vi "Auth Async.vi"(4 "Failed Response":refnum<class "Response.lvclass">, 6 "Complete Response":refnum<class "Response.lvclass">, 7 "Refresh Only?":bool, 9 "Timeout S":dbl=60.0, 10 "Async Authorization":refnum<class "Async Authorization.lvclass">, 11 "OAuth2 in":refnum<class "OAuth2.lvclass">) -> ()   [LabVIEW 2020, in "OAuth2.lvlib" / "OAuth2.lvclass"]
uses:
  OAuth2.lvclass
  OAuth2.lvclass/OAuth2.ctl
  Async Auth State.ctl
  OAuth2.lvlib
  lv-http-util/HTTP Utils/Request/Request.lvclass
  Async Authorization/Async Authorization.lvclass
  Request/Request.lvclass
  <vilib>/httpClient/LabVIEWHTTPClient.lvlib
  <vilib>/httpClient/POSTBuffer.vi
  lv-http-util/HTTP Utils/Response/Response.lvclass
  <vilib>/Platform/browser.llb/Open URL in Default Browser (string).vi
panel:
  out "Request URL":string
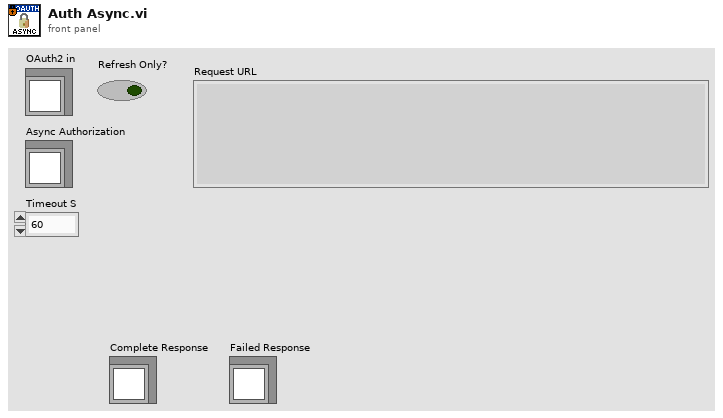
[diagram p1: front panel]
types:
  T1 = typedef "OAuth2.lvlib/Async Auth State.ctl" = enum16{"Initialize", "Request", "WaitAuth", "GetToken", "RefreshToken", "Complete", "Failed"}
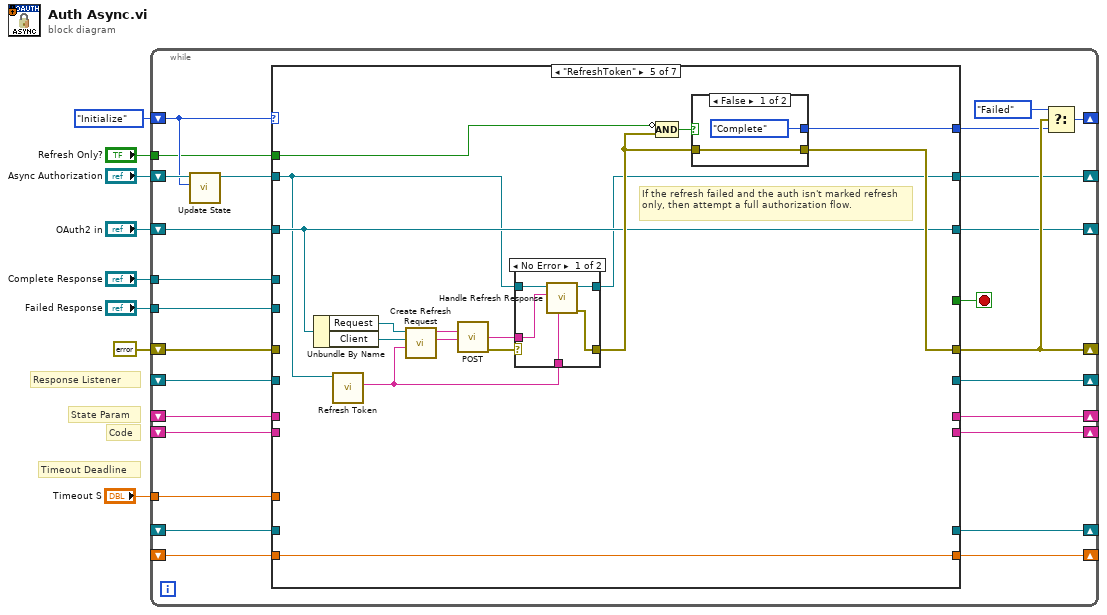
[diagram p0: block diagram]
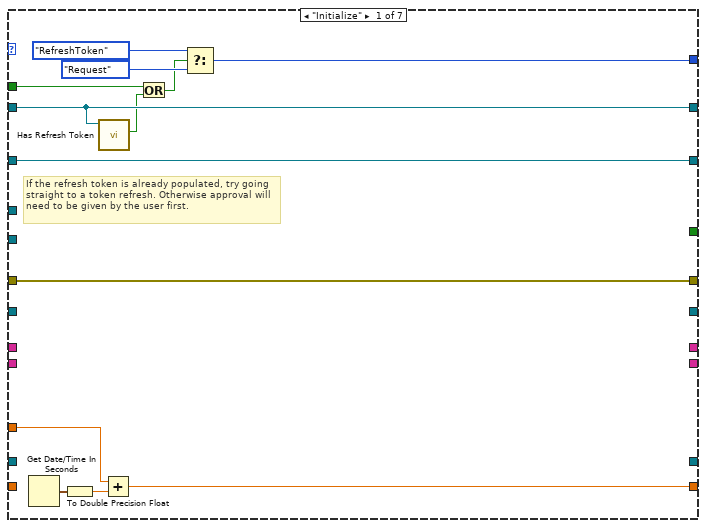
[diagram p2: hidden frame]
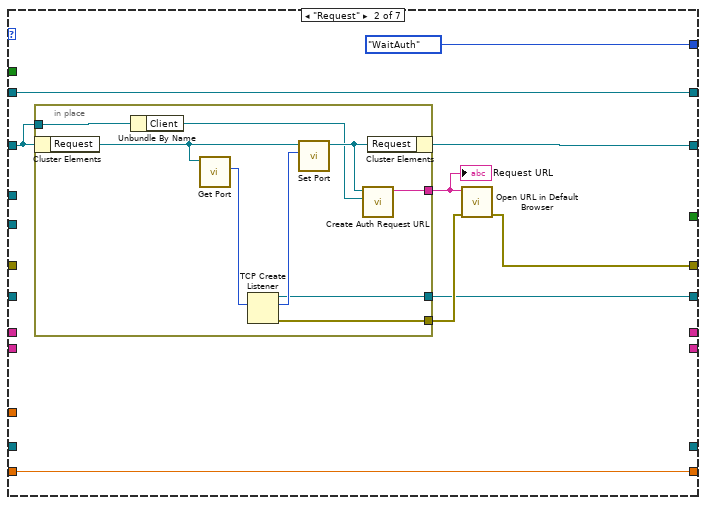
[diagram p3: hidden frame]
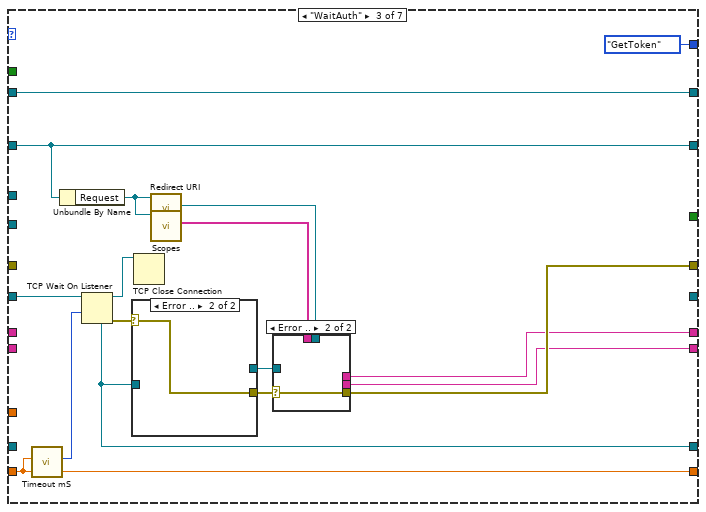
[diagram p4: hidden frame]
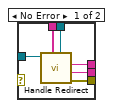
[diagram p5: hidden frame]
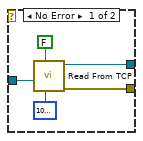
[diagram p6: hidden frame]
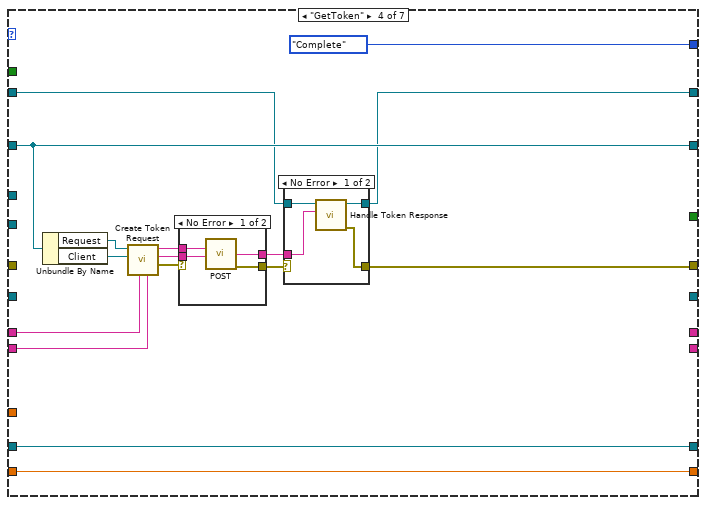
[diagram p7: hidden frame]
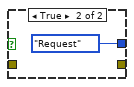
[diagram p10: hidden frame]
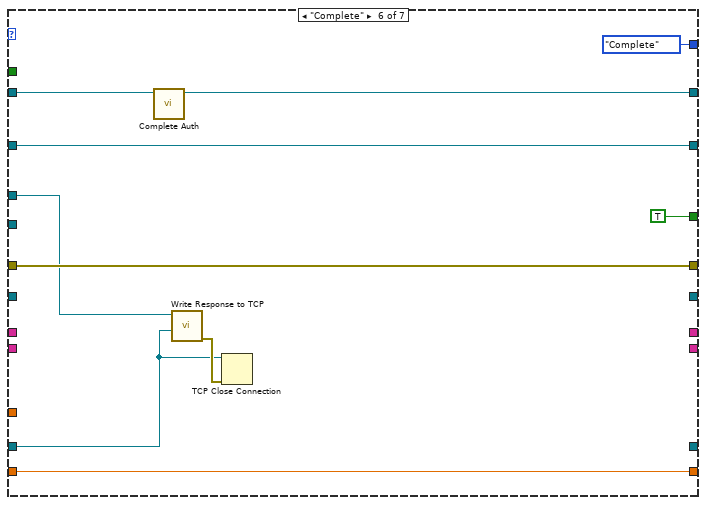
[diagram p12: hidden frame]
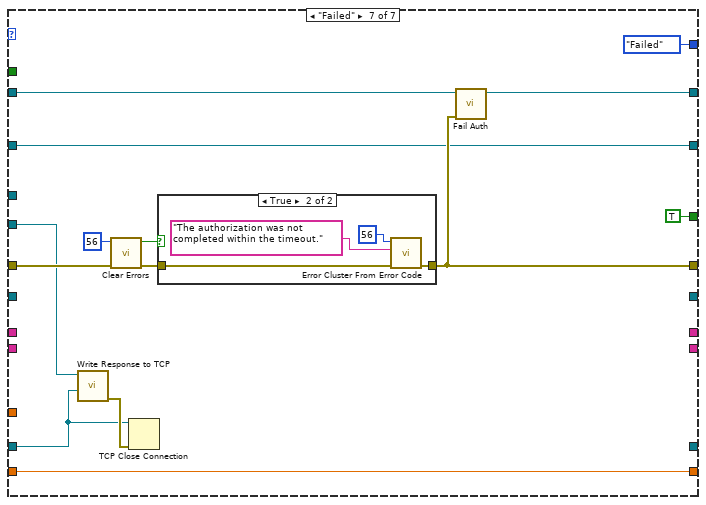
[diagram p13: hidden frame]
diagram:
  # "Timeout Deadline"
  # "Code"
  # "State Param"
  # "Response Listener"
  n1 = while {
    shift-right: [w18] -> _
    shift-left: Async_Auth_State."Initialize" ("State") -> [w28]
    shift-right: [w32] -> _
    shift-left: "OAuth2 in" -> [w33]
    shift-right: [w27] -> _
    shift-left: _ -> [w31]
    shift-right: [w26] -> _
    shift-left: _ -> [w24]
    shift-right: [w25] -> _
    shift-left: _ -> [w23]
    tunnel: "Timeout S" -> [w22]
    shift-right: [w21] -> _
    shift-left: _ -> [w20]
    shift-right: [w34] -> _
    shift-left: errorcluster {"status"=FALSE, "code"=0, "source"=""} ("error out") -> [w19]
    shift-right: [w15] -> _
    shift-left: "Async Authorization" -> [w30]
    tunnel: "Complete Response" -> [w13]
    tunnel: "Failed Response" -> [w12]
    shift-right: [w11] -> _
    shift-left: _ -> [w10]
    tunnel: "Refresh Only?" -> [w9]
    stop <- w14 stop-if-true
    n2 = call "Update State.vi"("Async Auth State"=w28, "Async Authorization in"=w30) -> ("Async Authorization out"=w29:refnum<class "Async Authorization.lvclass">)  [unwired: 9 in]
    n3 = case shown="\"RefreshToken\"" w28 {
      tunnel: w33 -> [w47 w54 w69 w111 w133 w152 w169]
      tunnel: [w47 w52 w69 w111 w133 w152 w169] -> w32
      tunnel: w31 -> [_ _ w81 _ _ _ _]
      tunnel: w29 -> [w39 w48 w76 w97 w127 w153 w167]
      tunnel: [_ w55 _ _ _ _ _] -> w27
      tunnel: [_ _ w71 _ _ _ _] -> w26
      tunnel: [_ _ w70 _ _ _ _] -> w25
      tunnel: w24 -> [_ _ _ w108 _ _ _]
      tunnel: w23 -> [_ _ _ w107 _ _ _]
      tunnel: w22 -> [w42 _ _ _ _ _ _]
      tunnel: [w41 w50 w80 w103 w136 w157 w168] -> w21
      tunnel: w20 -> [_ w50 w80 w103 w136 w157 w168]
      tunnel: [w38 w51 w72 w100 w138 w155 w171] -> w34
      tunnel: w19 -> [w38 _ _ _ _ w155 w172]
      tunnel: [w40 Async_Auth_State."WaitAuth" ("State") Async_Auth_State."GetToken" ("f") Async_Auth_State."Complete" ("f") w124 Async_Auth_State."Complete" ("f") Async_Auth_State."Failed" ("f")] -> w16
      tunnel: [w39 w48 w76 w98 w128 w151 w166] -> w15
      tunnel: [_ _ _ _ _ TRUE TRUE] -> w14
      tunnel: w13 -> [_ _ _ _ _ w149 _]
      tunnel: w12 -> [_ _ _ _ _ _ w163]
      tunnel: [_ _ w75 w96 _ _ _] -> w11
      tunnel: w10 -> [_ _ _ w96 _ w150 w162]
      tunnel: w9 -> [w37 _ _ _ w125 _ _]
      frame "Initialize" {
        # "If the refresh token is already populated, try going straight to a token refresh. Otherwise approval will need to be given by the user first."
        n4 = Get Date/Time In Seconds() -> (seconds since 1Jan1904=w44:timestamp)
        n5 = To Double Precision Float(number=w44) -> (double precision float=w43:dbl)
        n6 = call "Has Refresh Token.vi"("Async Authorization in"=w39) -> ("Has Refresh Token"=w36:bool)  [unwired: 10 in]
        n7 = Add(x=w42, y=w43) -> (x+y=w41:dbl)
        n8 = Or(x=w37, y=w36) -> (x .or. y?=w35:bool)
        n9 = Select(t=Async_Auth_State."RefreshToken" ("State"), s=w35, f=Async_Auth_State."Request") -> (s? t:f=w40:T1)
      }
      frame "Request" {
        n10 = in-place {
          in-place-border: [w63] -> w55
          in-place-border: w54 -> [w62]
          in-place-border: [w59] -> w53
          in-place-border: [w58] -> w56
          n11 = in-place-cluster #1(w54) -> ("Request"=w57:refnum<class "Request.lvclass">)
          n12 = Unbundle By Name(w62) -> ("Client"=w60:refnum<class "Client.lvclass">)
          n13 = call "Get Port.vi"("Request in"=w57) -> ("Port"=w65:u16)  [unwired: 10 in]
          n14 = TCP Create Listener(10:w65) -> (0:w58:errorcluster, 2:w64:u16, 3:w63:refnum<k5>)  [unwired: 4 in]
          n15 = call "Set Port.vi"("Port"=w64, "Request in"=w57) -> ("Request out"=w61:refnum<class "Request.lvclass">)  [unwired: 9 in]
          n16 = call "Create Auth Request URL.vi"("Client"=w60, "Request in"=w61) -> ("Request URL"=w59:string)  [unwired: 9 in]
          n17 = in-place-cluster #1("Request"=w61) -> (w52:refnum<class "OAuth2.lvclass">)
        }
        "Request URL" <- w53
        n18 = call-poly <vilib>:"Open URL in Default Browser.vi"("error in (no error)"=w56, "URL"=w53) -> ("error out"=w51:errorcluster)  [unwired: 4 in, 1 out]
      }
      frame "WaitAuth" {
        n19 = call "Timeout mS.vi"("Deadline"=w80) -> ("Timeout mS"=w79:i32)  [unwired: 10 in]
        n20 = Unbundle By Name(w69) -> ("Request"=w67:refnum<class "Request.lvclass">)
        n21 = TCP Wait On Listener(9:w79, 11:w81) -> (0:w82:errorcluster, 3:w78:refnum<k5>, 4:w75:refnum<k5>)  [unwired: 2 in, 2 out]
        n22 = case shown="Error .." w82 {
          selector: w82 -> [_ w95]
          tunnel: w75 -> [w90 _]
          tunnel: [w94 w95] -> w74
          tunnel: [w91 _] -> w73
          frame No Error {
            n23 = call "Read From TCP.vi"("Max Size (50MB)"=u64 1000000, "Uploads as Files? (T)"=FALSE, "TCP Connection"=w90) -> ("error out"=w94:errorcluster, "Request out"=w91:refnum<class "Request.lvclass">)  [unwired: 7 in]
          }
          frame Error {
          }
        }
        n24 = TCP Close Connection(connection ID=w78) -> ()  [unwired: 2 in, 2 out]
        n25 = call "Redirect URI.vi"("Request in"=w67) -> ("Redirect URI"=w66:refnum<class "URI.lvclass">)  [unwired: 10 in]
        n26 = call "Scopes.vi"("Request in"=w67) -> ("Scopes"=w68:string[])  [unwired: 10 in]
        n27 = case shown="Error .." w74 {
          selector: w74 -> [_ w89]
          tunnel: w73 -> [w88 _]
          tunnel: [w87 w89] -> w72
          tunnel: [w86 _] -> w71
          tunnel: [w85 _] -> w70
          tunnel: w68 -> [w84 _]
          tunnel: w66 -> [w83 _]
          frame No Error {
            n28 = call "Handle Redirect.vi"("Redirect URI"=w83, "Requested Scopes"=w84, "Request in"=w88) -> ("error out"=w87:errorcluster, "Code"=w85:string, "State Param"=w86:string)  [unwired: 6 in]
          }
          frame Error {
          }
        }
      }
      frame "GetToken" {
        n29 = Unbundle By Name(w111) -> ("Request"=w110:refnum<class "Request.lvclass">, "Client"=w109:refnum<class "Client.lvclass">)
        n30 = call "Create Token Request.vi"("Code"=w107, "State"=w108, "Client"=w109, "Request in"=w110) -> ("error out"=w106:errorcluster, "POST Buffer"=w105:string, "Request URL"=w104:string)  [unwired: 5 in]
        n31 = case shown="No Error" w106 {
          selector: w106 -> [_ w122]
          tunnel: w105 -> [w120 _]
          tunnel: w104 -> [w121 _]
          tunnel: [w119 w122] -> w102
          tunnel: [w118 _] -> w101
          frame No Error {
            n32 = call-poly <vilib>:"POST.vi"("url"=w121, "buffer"=w120) -> ("body"=w118:string, "error out"=w119:errorcluster)  [unwired: 10 in, 2 out]
          }
          frame Error {
          }
        }
        n33 = case shown="No Error" w102 {
          selector: w102 -> [_ w117]
          tunnel: w101 -> [w114 _]
          tunnel: w97 -> [w115 w116]
          tunnel: [w113 w117] -> w100
          tunnel: [w112 w116] -> w98
          frame No Error {
            n34 = call "Handle Token Response.vi"("Response Body"=w114, "Async Authorization in"=w115) -> ("error out"=w113:errorcluster, "Asyn Authorization out"=w112:refnum<class "Async Authorization.lvclass">)  [unwired: 8 in]
          }
          frame Error {
          }
        }
      }
      frame "RefreshToken" {
        # "If the refresh failed and the auth isn't marked refresh only, then attempt a full authorization flow."
        n35 = Unbundle By Name(w133) -> ("Request"=w131:refnum<class "Request.lvclass">, "Client"=w132:refnum<class "Client.lvclass">)
        n36 = call "Refresh Token.vi"("Async Authorization in"=w127) -> ("Refresh Token"=w126:string)  [unwired: 10 in]
        n37 = call "Create Refresh Request.vi"("Refresh Token"=w126, "Client"=w132, "Request in"=w131) -> ("POST Buffer"=w129:string, "Request URL"=w130:string)  [unwired: 7 in]
        n38 = call-poly <vilib>:"POST.vi"("url"=w130, "buffer"=w129) -> ("body"=w134:string, "error out"=w135:errorcluster)  [unwired: 10 in, 2 out]
        n39 = case shown="No Error" w135 {
          selector: w135 -> [_ w148]
          tunnel: w134 -> [w145 _]
          tunnel: w127 -> [w146 w147]
          tunnel: [w144 w148] -> w137
          tunnel: [w143 w147] -> w128
          tunnel: w126 -> [w142 _]
          frame No Error {
            n40 = call "Handle Refresh Response.vi"("Refresh Token"=w142, "Response Body"=w145, "Async Authorization in"=w146) -> ("error out"=w144:errorcluster, "Asyn Authorization out"=w143:refnum<class "Async Authorization.lvclass">)  [unwired: 7 in]
          }
          frame Error {
          }
        }
        n41 = Compound Arithmetic op=AND(invert w125, w137) -> (w123:bool)
        n42 = case shown="False" w123 {
          tunnel: [Async_Auth_State."Complete" ("f") Async_Auth_State."Request" ("f")] -> w124
          tunnel: w137 -> [w139 _]
          tunnel: [w139 _] -> w138
          frame False {
          }
          frame True {
          }
        }
      }
      frame "Complete" {
        (unwired) TRUE
        n43 = call "Complete Auth.vi"("Async Authorization in"=w153) -> ("Async Authorization out"=w151:refnum<class "Async Authorization.lvclass">)  [unwired: 9 in, 1 out]
        n44 = call "Write Response to TCP.vi"("TCP Connection"=w150, "Response in"=w149) -> ("error out"=w158:errorcluster)  [unwired: 8 in, 1 out]
        n45 = TCP Close Connection(connection ID=w150, error in (no error)=w158) -> ()  [unwired: 1 in, 2 out]
      }
      frame "Failed" {
        (unwired) TRUE
        n46 = call "Write Response to TCP.vi"("TCP Connection"=w162, "Response in"=w163) -> ("error out"=w170:errorcluster)  [unwired: 8 in, 1 out]
        n47 = call <vilib>:"Clear Errors.vi"("error in (no error)"=w172, "specific error code to clear (0: all)"=56) -> ("error out"=w160:errorcluster, "specific error cleared?"=w159:bool)  [unwired: 4 in]
        n48 = TCP Close Connection(connection ID=w162, error in (no error)=w170) -> ()  [unwired: 1 in, 2 out]
        n49 = case shown="True" w159 {
          tunnel: w160 -> [w173 w177]
          tunnel: [w173 w175] -> w171
          frame False {
          }
          frame True {
            n50 = call <vilib>:"Error Cluster From Error Code.vi"("error in (no error)"=w177, "error message (\"\")"="The authorization was not completed within the timeout." ("error message (\"\")"), "error code (0)"=56) -> ("error out"=w175:errorcluster)  [unwired: 6 in]
          }
        }
        n51 = call "Fail Auth.vi"("error in (no error)"=w171, "Async Authorization in"=w167) -> ("Async Authorization out"=w166:refnum<class "Async Authorization.lvclass">)  [unwired: 8 in, 1 out]
      }
    }
    n52 = Select(t=Async_Auth_State."Failed" ("State"), s=w34, f=w16) -> (s? t:f=w18:T1)
  }
